vi "Write Data by Creating New File.vi"() -> ()   [LabVIEW 2016]
panel:
  in  "Data":string
  in  "Operation on File":T1(ring)
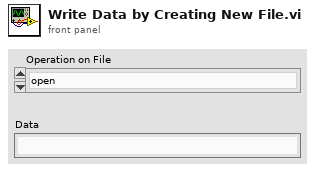
[diagram p1: front panel]
types:
  T1 = enum16{"open", "replace", "create", "open or create", "replace or create", "replace or create with confirmation"}
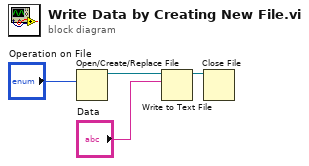
[diagram p0: block diagram]
diagram:
  n1 = Open/Create/Replace File(operation (0:open)="Operation on File") -> (refnum out=w4:refnum<file>)  [unwired: 5 in, 2 out]
  n2 = Write to Text File(file (use dialog)=w4, text="Data") -> (refnum out=w3:refnum<file>)  [unwired: 2 in, 2 out]
  n3 = Close File(refnum=w3) -> ()  [unwired: 1 in, 2 out]
